vi "New MemberController.vi"(6 "Database":refnum<class "Database.lvclass">, 8 "error in (no error)":errorcluster, 9 "Name('')":string, 10 "ID(\"\")":string, 11 "Member_Actor in":refnum<class "Member_Actor.lvclass">) -> (0 "error out":errorcluster, 3 "Member_Actor out":refnum<class "Member_Actor.lvclass">)   [LabVIEW 2015, in "Member_Actor.lvlib" / "Member_Actor.lvclass"]
uses:
  Member_Actor.lvclass
  API/_Database/Database.lvclass
  Member_Actor.lvclass/Member_Actor.ctl
  Admin_Actor/Setting/g_setting.vi
  Admin_Actor/Admin_Actor.lvlib
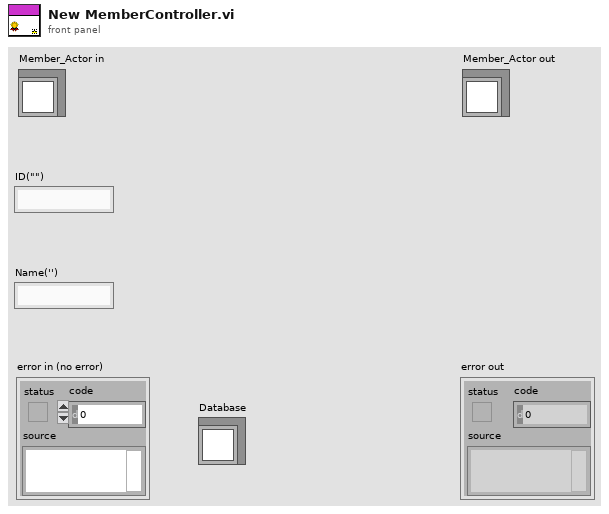
[diagram p1: front panel]
types:
  T1 = typedef "LVDateTimeRec.ctl" = cluster{"fractional second":dbl, "second":i32, "minute":i32, "hour":i32, "day of month":i32, "month":i32, "year":i32, "day of week":i32, "day of year":i32, "DST":i32}
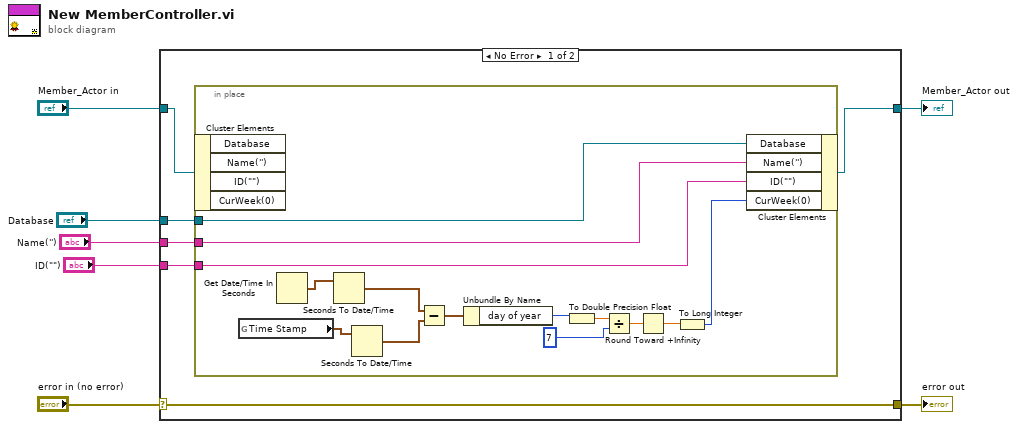
[diagram p0: block diagram]
diagram:
  n1 = case shown="No Error" "error in (no error)" {
    selector: "error in (no error)" -> [w13 w29]
    tunnel: [w13 w29] -> w6
    tunnel: [w8 w28] -> w4
    tunnel: "Member_Actor in" -> [w12 w28]
    tunnel: "ID(\"\")" -> [w11 _]
    tunnel: "Name('')" -> [w10 _]
    tunnel: "Database" -> [w9 _]
    frame No Error {
      n2 = in-place {
        in-place-border: w11 -> [w16]
        in-place-border: w10 -> [w15]
        in-place-border: w9 -> [w14]
        n3 = in-place-cluster #1(w12) -> ()  [unwired: 4 out]
        n4 = global read "g_setting.vi" "Time Stamp"() -> (w26:timestamp)
        n5 = Get Date/Time In Seconds() -> (seconds since 1Jan1904=w27:timestamp)
        n6 = Seconds To Date/Time(time stamp (now)=w27) -> (date time rec=w25:T1)  [unwired: 1 in]
        n7 = Seconds To Date/Time(time stamp (now)=w26) -> (date time rec=w24:T1)  [unwired: 1 in]
        n8 = Subtract(x=w25, y=w24) -> (x-y=w23:T1)
        n9 = Unbundle By Name(w23) -> ("day of year"=w22:i32)
        n10 = To Double Precision Float(number=w22) -> (double precision float=w21:dbl)
        n11 = Divide(x=w21, y=7) -> (x/y=w19:dbl)
        n12 = Round Toward +Infinity(x=w19) -> (ceil(x): smallest int >= x=w18:dbl)
        n13 = To Long Integer(number=w18) -> (32bit integer=w17:i32)
        n14 = in-place-cluster #1("Database"=w14, "Name('')"=w15, "ID(\"\")"=w16, "CurWeek(0)"=w17) -> (w8:refnum<class "Member_Actor.lvclass">)
      }
    }
    frame Error {
    }
  }
  "error out" <- w6
  "Member_Actor out" <- w4
